vi "FDL.vi"(0 "System no.":i32=1 min=1 step=1, 2 "Routinename":string, 3 "Scan axis settings":T2={"Scan axis"="", "Range scan axis"=0.1, "Mid. pos. scan axis"=0.0, "Calc. pos. scan axis"=0.0} {"Calc. pos. scan axis" format="%.4f"; "Mid. pos. scan axis" format="%.4f"; "Range scan axis" format="%.4f"}, 4 "Step axis settings":T1={"Step axis"="", "Range step axis"=0.1, "Mid. pos. step axis"=0.0, "Calc. pos. step axis"=0.0} {"Calc. pos. step axis" format="%.4f"; "Mid. pos. step axis" format="%.4f"; "Range step axis" format="%.4f"}, 5 "error in":errorcluster, 6 "Minimum threshold settings":cluster{"Threshold sigma":i32}={"Threshold sigma"=100}, 7 "Alignment input channel settings":cluster{"Alignment signal input channel":i32}={"Alignment signal input channel"=1}, 8 "Threshold calculation settings":cluster{"Threshold calculation":bool}={"Threshold calculation"=TRUE}, 9 "Search time settings":cluster{"Maximum search time [s]":dbl}={"Maximum search time [s]"=5.0} {"Maximum search time [s]" format="%.4f"}) -> (19 "error out":errorcluster)   [LabVIEW 2026]
doc: "Defines a \"PILightning\" scan, a fast alignment scan routine for first light search. For a detailed description, see the Technical Note E712T0016 (\"Fast Alignment Routines\")."
panel:
  # "Defines a fast alignment scan routine for first light search, also refererred to as\n\"PILightning scan\". Use FRS to start the routine and FRR? to read out the results of the routine."
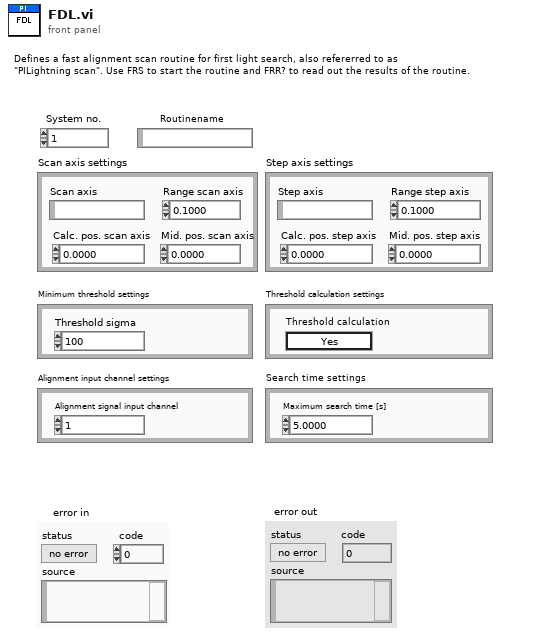
[diagram p1: front panel]
types:
  T1 = cluster{"Step axis":string, "Range step axis":dbl, "Mid. pos. step axis":dbl, "Calc. pos. step axis":dbl}
  T2 = cluster{"Scan axis":string, "Range scan axis":dbl, "Mid. pos. scan axis":dbl, "Calc. pos. scan axis":dbl}
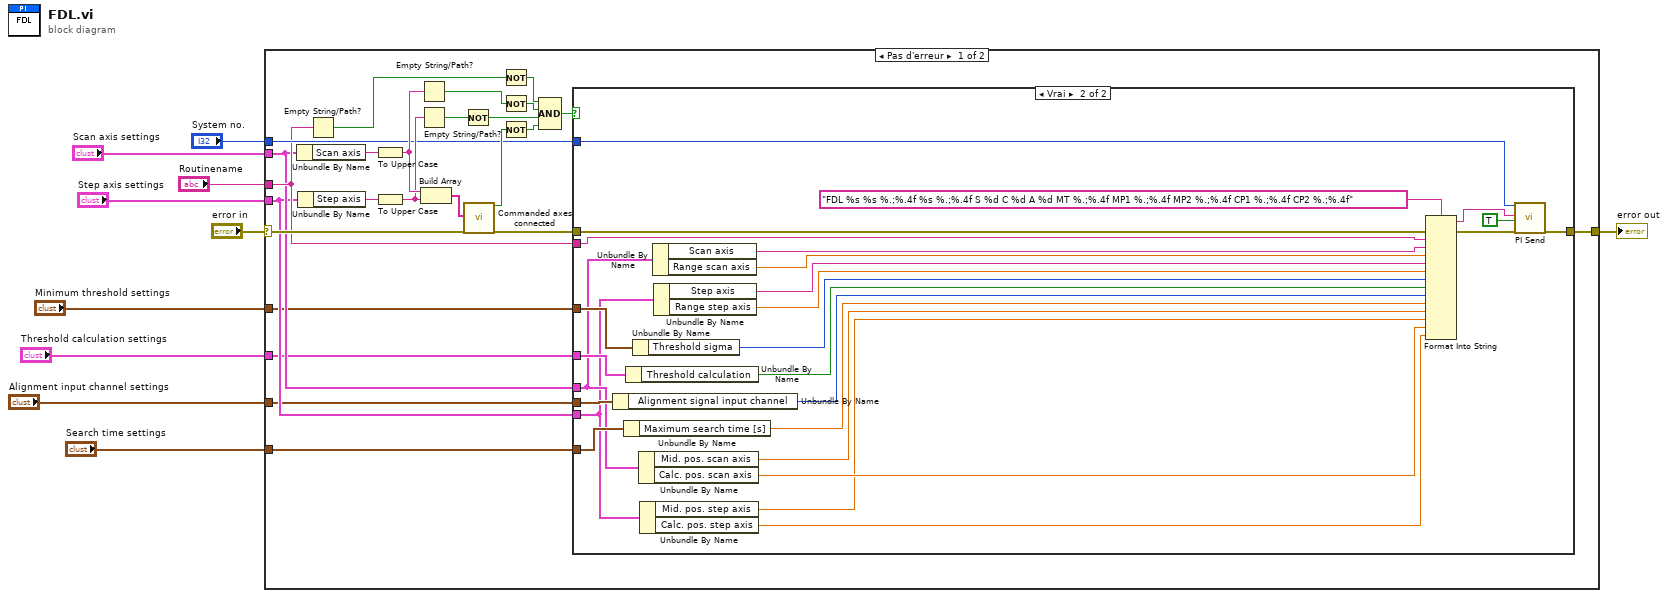
[diagram p0: block diagram]
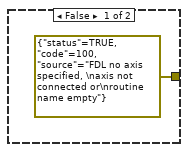
[diagram p2: hidden frame]
diagram:
  n1 = case shown="Pas d'erreur" "error in" {
    selector: "error in" -> [w31 w63]
    tunnel: [w20 w63] -> w9
    tunnel: "System no." -> [w18 _]
    tunnel: "Routinename" -> [w17 _]
    tunnel: "Scan axis settings" -> [w16 _]
    tunnel: "Step axis settings" -> [w15 _]
    tunnel: "Threshold calculation settings" -> [w11 _]
    tunnel: "Minimum threshold settings" -> [w14 _]
    tunnel: "Search time settings" -> [w13 _]
    tunnel: "Alignment input channel settings" -> [w12 _]
    frame No Error {
      n2 = Unbundle By Name(w16) -> ("Scan axis"=w33:string)
      n3 = Unbundle By Name(w15) -> ("Step axis"=w32:string)
      n4 = Empty String/Path?(string/path=w17) -> (empty?=w30:bool)
      n5 = To Upper Case(1:w33) -> (0:w27:string)
      n6 = To Upper Case(1:w32) -> (0:w26:string)
      n7 = Empty String/Path?(string/path=w27) -> (empty?=w29:bool)
      n8 = Empty String/Path?(string/path=w26) -> (empty?=w28:bool)
      n9 = Build Array(w27, w26) -> (w35:string[])
      n10 = Not(x=w28) -> (.not. x?=w24:bool)
      n11 = call "Commanded axes connected.vi"("Commanded axes"=w35, "error in"=w31) -> ("Controller error"=w34:bool, "error out"=w21:errorcluster)  [unwired: 1 in, 15 out]
      n12 = Not(x=w30) -> (.not. x?=w19:bool)
      n13 = Not(x=w29) -> (.not. x?=w25:bool)
      n14 = Not(x=w34) -> (.not. x?=w23:bool)
      n15 = Compound Arithmetic op=AND(w19, w25, w24, w23) -> (w22:bool)
      n16 = case shown="Vrai" w22 {
        tunnel: w21 -> [_ w55]
        tunnel: [errorcluster {"status"=TRUE, "code"=100, "source"="FDL no axis specified, \naxis not connected or\nroutine name empty"} ("error out") w60] -> w20
        tunnel: w18 -> [_ w59]
        tunnel: w17 -> [_ w56]
        tunnel: w16 -> [_ w42]
        tunnel: w15 -> [_ w39]
        tunnel: w14 -> [_ w50]
        tunnel: w13 -> [_ w44]
        tunnel: w12 -> [_ w48]
        tunnel: w11 -> [_ w47]
        frame False {
        }
        frame True {
          n17 = Unbundle By Name(w48) -> ("Alignment signal input channel"=w45:i32)
          n18 = Unbundle By Name(w44) -> ("Maximum search time [s]"=w43:dbl)
          n19 = Unbundle By Name(w47) -> ("Threshold calculation"=w46:bool)
          n20 = Unbundle By Name(w50) -> ("Threshold sigma"=w49:i32)
          n21 = Unbundle By Name(w42) -> ("Mid. pos. scan axis"=w41:dbl, "Calc. pos. scan axis"=w40:dbl)
          n22 = Unbundle By Name(w39) -> ("Mid. pos. step axis"=w38:dbl, "Calc. pos. step axis"=w37:dbl)
          n23 = Unbundle By Name(w42) -> ("Scan axis"=w57:string, "Range scan axis"=w53:dbl)
          n24 = Unbundle By Name(w39) -> ("Step axis"=w52:string, "Range step axis"=w51:dbl)
          n25 = Format Into String(format string="FDL %s %s %.;%.4f %s %.;%.4f S %d C %d A %d MT %.;%.4f MP1 %.;%.4f MP2 %.;%.4f CP1 %.;%.4f CP2 %.;%.4f" ("Format String"), error in=w55, w56, w57, w53, w52, w51, w49, w46, w45, w43, w41, w38, w40, w37) -> (resulting string=w58:string, error out=w54:errorcluster)  [unwired: 1 in]
          n26 = call "PI Send.vi"("System no."=w59, "String to send"=w58, "Attach termination char.?"=TRUE, "error in"=w54) -> ("error out"=w60:errorcluster)  [unwired: 2 in, 13 out]
        }
      }
    }
    frame Error {
    }
  }
  "error out" <- w9
